vi "dfd_MRate Single Block Preprocessing.vi"(6 "zerophase ?":bool=TRUE, 8 "error in (no error)":errorcluster, 9 "extension type":u16(ring) items=["zero padding", "symmetric", "periodic"], 10 "multirate filter in":T1={"mMRate_Structure"=enum."CIC", "mMRate_Mode"=0, "mMRate_Factor"=1, "mMRate_FIRParams"={"mMRate_FIR_H"=[], "mMRate_FIR_IsNyquist?"=FALSE, "mMRate_FIR_IsSymmetric?"=FALSE}, "mMRate_CICParams"={"mMRate_CIC_#Stage"=2, "mMRate_CIC_Lag"=1, "mMRate_CIC_Type"=enum."Lowpass"}, "mMRate_Order"=1, "mMRate_Version"="1.0", "mMRate_Comments"="1.0", "mMRate_RationalFactor"={"mMRate_L"=-1, "mMRate_M"=-1}, "mMRate_Fs"=1.0, "mMRate_Quantized?"=FALSE, "mMRate_QFilterGain"=1.0, "mMRate_CoefWl"=16, "mMRate_Scaling"={"mMRate_ScaleByPowerOf2?"=FALSE, "mMRate_ScaleType"=enum."Time Domain 1-Norm"}, "mMRate_InputWl"=0, "mMRate_OutputWl"=0, "mMRate_OutputMode"=enum."Nearest", "mMRate_MultMode"=enum."Full", "mMRate_BitPruning"=FALSE, "mMRate_GainWl"=16, "mMRate_OutputFwl"=0, "mMRate_SumIwl"=0, "mMRate_InputIwl "=16, "mMRate_SumWl"=32, "mMRate_CoefIwl"=0} {"mMRate_SumWl" min=1 max=32 step=1; "mMRate_InputIwl" min=1 max=32 step=1; "mMRate_GainWl" min=1 max=32 step=1; "mMRate_OutputWl" min=1 max=32 step=1; "mMRate_InputWl" min=1 max=32 step=1; "mMRate_CoefWl" min=1 max=32 step=1; "mMRate_Mode" items=["Default"=-1, "No Rate Change"=0, "Interpolation"=1, "Decimation"=2, "Interpolated"=3, "Rational"=4]}, 11 "x":dbl[](array[numeric])) -> (0 "error out":errorcluster, 2 "dup multirate filter":T1={"mMRate_Structure"=enum."CIC", "mMRate_Mode"=0, "mMRate_Factor"=1, "mMRate_FIRParams"={"mMRate_FIR_H"=[], "mMRate_FIR_IsNyquist?"=FALSE, "mMRate_FIR_IsSymmetric?"=FALSE}, "mMRate_CICParams"={"mMRate_CIC_#Stage"=2, "mMRate_CIC_Lag"=1, "mMRate_CIC_Type"=enum."Lowpass"}, "mMRate_Order"=1, "mMRate_Version"="1.0", "mMRate_Comments"="1.0", "mMRate_RationalFactor"={"mMRate_L"=-1, "mMRate_M"=-1}, "mMRate_Fs"=1.0, "mMRate_Quantized?"=FALSE, "mMRate_QFilterGain"=1.0, "mMRate_CoefWl"=16, "mMRate_Scaling"={"mMRate_ScaleByPowerOf2?"=FALSE, "mMRate_ScaleType"=enum."Time Domain 1-Norm"}, "mMRate_InputWl"=0, "mMRate_OutputWl"=0, "mMRate_OutputMode"=enum."Nearest", "mMRate_MultMode"=enum."Full", "mMRate_BitPruning"=FALSE, "mMRate_GainWl"=16, "mMRate_OutputFwl"=0, "mMRate_SumIwl"=0, "mMRate_InputIwl "=16, "mMRate_SumWl"=32, "mMRate_CoefIwl"=0} {"mMRate_SumWl" min=1 max=32 step=1; "mMRate_InputIwl" min=1 max=32 step=1; "mMRate_GainWl" min=1 max=32 step=1; "mMRate_OutputWl" min=1 max=32 step=1; "mMRate_InputWl" min=1 max=32 step=1; "mMRate_CoefWl" min=1 max=32 step=1; "mMRate_Mode" items=["Default"=-1, "No Rate Change"=0, "Interpolation"=1, "Decimation"=2, "Interpolated"=3, "Rational"=4]}, 3 "y":dbl[](array[numeric]), 4 "output phase":i32, 5 "output length":i32, 7 "pre cut length":i32)   [LabVIEW 2017, in "NI_DigFilter_Process.lvlib"]
uses:
  <vilib>/addons/Digital Filter Design/NI_DigFilter_Process.lvlib
  <vilib>/addons/Digital Filter Design/_Objects.llb/DFD Multirate Filter Obj.ctl
  <vilib>/addons/Digital Filter Design/_Objects.llb/DFD Multirate Mode.ctl
  <vilib>/addons/Digital Filter Design/_Objects.llb/DFD Coef Norm Type.ctl
  <vilib>/addons/Digital Filter Design/_Objects.llb/DFD Round-off Mode.ctl
  <vilib>/addons/Digital Filter Design/_Objects.llb/DFD FXP MRate Multiply Mode.ctl
  <vilib>/addons/Digital Filter Design/NI_DigFilterLicensed.lvlib
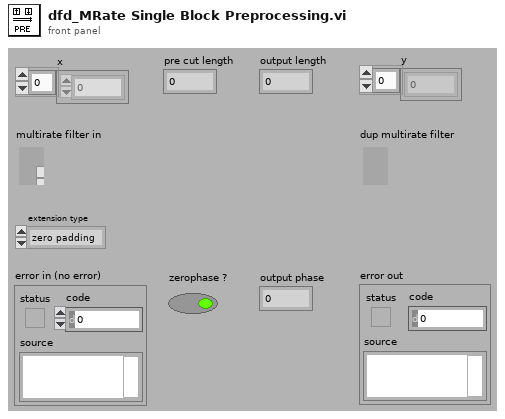
[diagram p1: front panel]
types:
  T1 = typedef "NI_DigFilterLicensed.lvlib/DFD Multirate Filter Obj.ctl" = cluster{"mMRate_Structure":enum16{"CIC", "FIR", "IIR", "Lattice"}, "mMRate_Mode":T2, "mMRate_Factor":i32, "mMRate_FIRParams":cluster{"mMRate_FIR_H":dbl[], "mMRate_FIR_IsNyquist?":bool, "mMRate_FIR_IsSymmetric?":bool}, "mMRate_CICParams":cluster{"mMRate_CIC_#Stage":i32, "mMRate_CIC_Lag":i32, "mMRate_CIC_Type":enum16{"Lowpass", "Highpass"}}, "mMRate_Order":i32, "mMRate_Version":string, "mMRate_Comments":string, "mMRate_RationalFactor":cluster{"mMRate_L":i32, "mMRate_M":i32}, "mMRate_Fs":dbl, "mMRate_Quantized?":bool, "mMRate_QFilterGain":dbl, "mMRate_CoefWl":i16, "mMRate_Scaling":cluster{"mMRate_ScaleByPowerOf2?":bool, "mMRate_ScaleType":T3}, "mMRate_InputWl":i16, "mMRate_OutputWl":i16, "mMRate_OutputMode":T4, "mMRate_MultMode":T5, "mMRate_BitPruning":bool, "mMRate_GainWl":i16, "mMRate_OutputFwl":i16, "mMRate_SumIwl":i16, "mMRate_InputIwl ":i16, "mMRate_SumWl":i16, "mMRate_CoefIwl":i16}
  T2 = typedef "NI_DigFilterLicensed.lvlib/DFD Multirate Mode.ctl" = i16
  T3 = typedef "NI_DigFilterLicensed.lvlib/DFD Coef Norm Type.ctl" = enum16{"No Norm", "Time Domain 1-Norm", "Time Domain 2-Norm", "Time Domain Inf-Norm"}
  T4 = typedef "NI_DigFilterLicensed.lvlib/DFD Round-off Mode.ctl" = enum16{"Nearest", "Truncation"}
  T5 = typedef "NI_DigFilterLicensed.lvlib/DFD FXP MRate Multiply Mode.ctl" = enum16{"Truncated", "Full"}
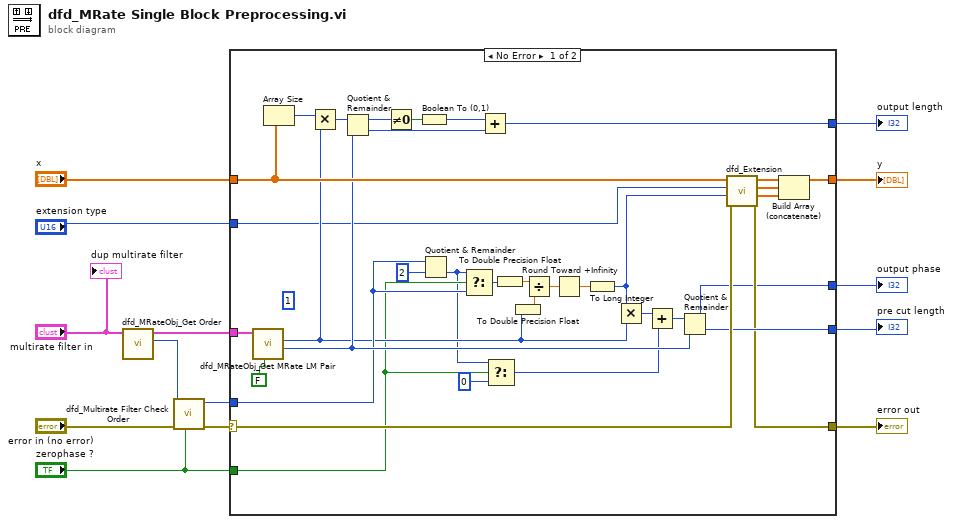
[diagram p0: block diagram]
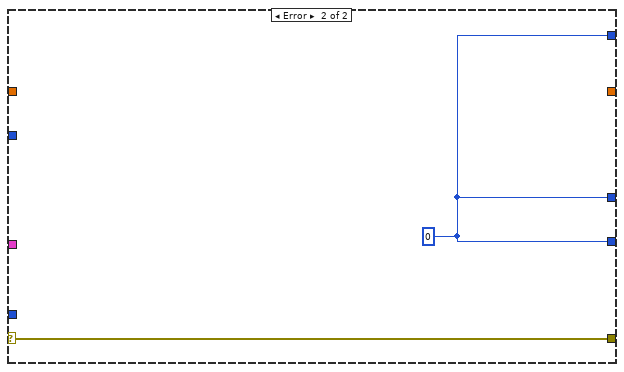
[diagram p2: hidden frame]
diagram:
  n1 = call <vilib>:"dfd_MRateObj_Get Order.vi"("multirate filter in"="multirate filter in") -> ("order"=w5:i32, "dup multirate filter"=w4:T1)  [unwired: 9 out]
  n2 = call <vilib>:"dfd_Multirate Filter Check Order.vi"("zeroPhase?"="zerophase ?", "error in (no error)"="error in (no error)", "order"=w5) -> ("error out"=w8:errorcluster, "dup order"=w7:i32)  [unwired: 7 out]
  n3 = case shown="No Error" w8 {
    selector: w8 -> [w48 w51]
    tunnel: [w46 w51] -> w14
    tunnel: [w49 _] -> w13
    tunnel: "extension type" -> [w17 _]
    tunnel: w4 -> [w44 _]
    tunnel: "x" -> [w43 _]
    tunnel: [w47 w50] -> w10
    tunnel: "zerophase ?" -> [w23 _]
    tunnel: w7 -> [w32 _]
    tunnel: [w26 w50] -> w6
    tunnel: [w45 w50] -> w2
    frame No Error {
      (unwired) 1
      n4 = call <vilib>:"dfd_MRateObj_Get MRate LM Pair.vi"("filter/fs (filter:T)"=FALSE, "multirate filter in"=w44) -> ("M"=w40:i32, "L"=w25:i32)  [unwired: 8 out]
      n5 = Array Size(array=w43) -> (size(s)=w41:i32)
      n6 = Multiply(x=w41, y=w25) -> (x*y=w42:i32)
      n7 = Quotient & Remainder(x=w42, y=w40) -> (x-y*floor(x/y)=w30:i32, floor(x/y)=w27:i32)
      n8 = Not Equal To 0?(x=w30) -> (x != 0?=w29:bool)
      n9 = Boolean To (0,1)(Boolean=w29) -> (0, 1=w28:i16)
      n10 = Quotient & Remainder(x=w32, y=2) -> (floor(x/y)=w22:i32)  [unwired: 1 out]
      n11 = Select(t=w22, s=w23, f=w32) -> (s? t:f=w31:i32)
      n12 = Add(x=w28, y=w27) -> (x+y=w26:i32)
      n13 = Select(t=w22, s=w23, f=0) -> (s? t:f=w20:i32)
      n14 = To Double Precision Float(number=w31) -> (double precision float=w15:dbl)
      n15 = To Double Precision Float(number=w25) -> (double precision float=w16:dbl)
      n16 = Divide(x=w15, y=w16) -> (x/y=w35:dbl)
      n17 = Round Toward +Infinity(x=w35) -> (ceil(x): smallest int >= x=w34:dbl)
      n18 = To Long Integer(number=w34) -> (32bit integer=w33:i32)
      n19 = Multiply(x=w33, y=w25) -> (x*y=w21:i32)
      n20 = Add(x=w21, y=w20) -> (x+y=w19:i32)
      n21 = Quotient & Remainder(x=w19, y=w40) -> (x-y*floor(x/y)=w45:i32, floor(x/y)=w47:i32)
      n22 = call <vilib>:"dfd_Extension.vi"("error in (no error)"=w48, "extension length"=w33, "extension type"=w17, "x[i]"=w43) -> ("error out"=w46:errorcluster, "final condition out"=w39:dbl[], "x[i] dup."=w37:dbl[], "initial condition out"=w38:dbl[])  [unwired: 4 out]
      n23 = Build Array (concatenate)(w38, w37, w39) -> (w49:dbl[])
    }
    frame Error {
      w50 = 0
    }
  }
  "pre cut length" <- w10
  "error out" <- w14
  "y" <- w13
  "output length" <- w6
  "output phase" <- w2
  "dup multirate filter" <- "multirate filter in"
